vi "time_all_in_one.vi"(8 "Error In":errorcluster, 9 "Ship data?":bool, 10 "controls":T3={"window duration"=1.0, "width"=5, "crossing level"=0.0, "threshold"=0.25, "Sec"=1.0, "start time"=0.0} {"start time" format="%#_13g"; "Sec" format="%0.2f"; "threshold" format="%0.2f"; "crossing level" format="%#_13g"; "width" min=3; "window duration" format="%0.2f"}, 11 "waveform in":waveform(dbl)) -> (0 "Error out":errorcluster, 3 "time data cluster":T2)   [LabVIEW 2020]
uses:
  <vilib>/Waveform/WDTOps.llb/WDT Get Waveform Subset DBL.vi
  <vilib>/Analysis/1siggen.llb/Ramp Pattern by Delta.vi
  <vilib>/Analysis/NI_AALBase.lvlib
panel:
  out "XY Graph":T1(graph)
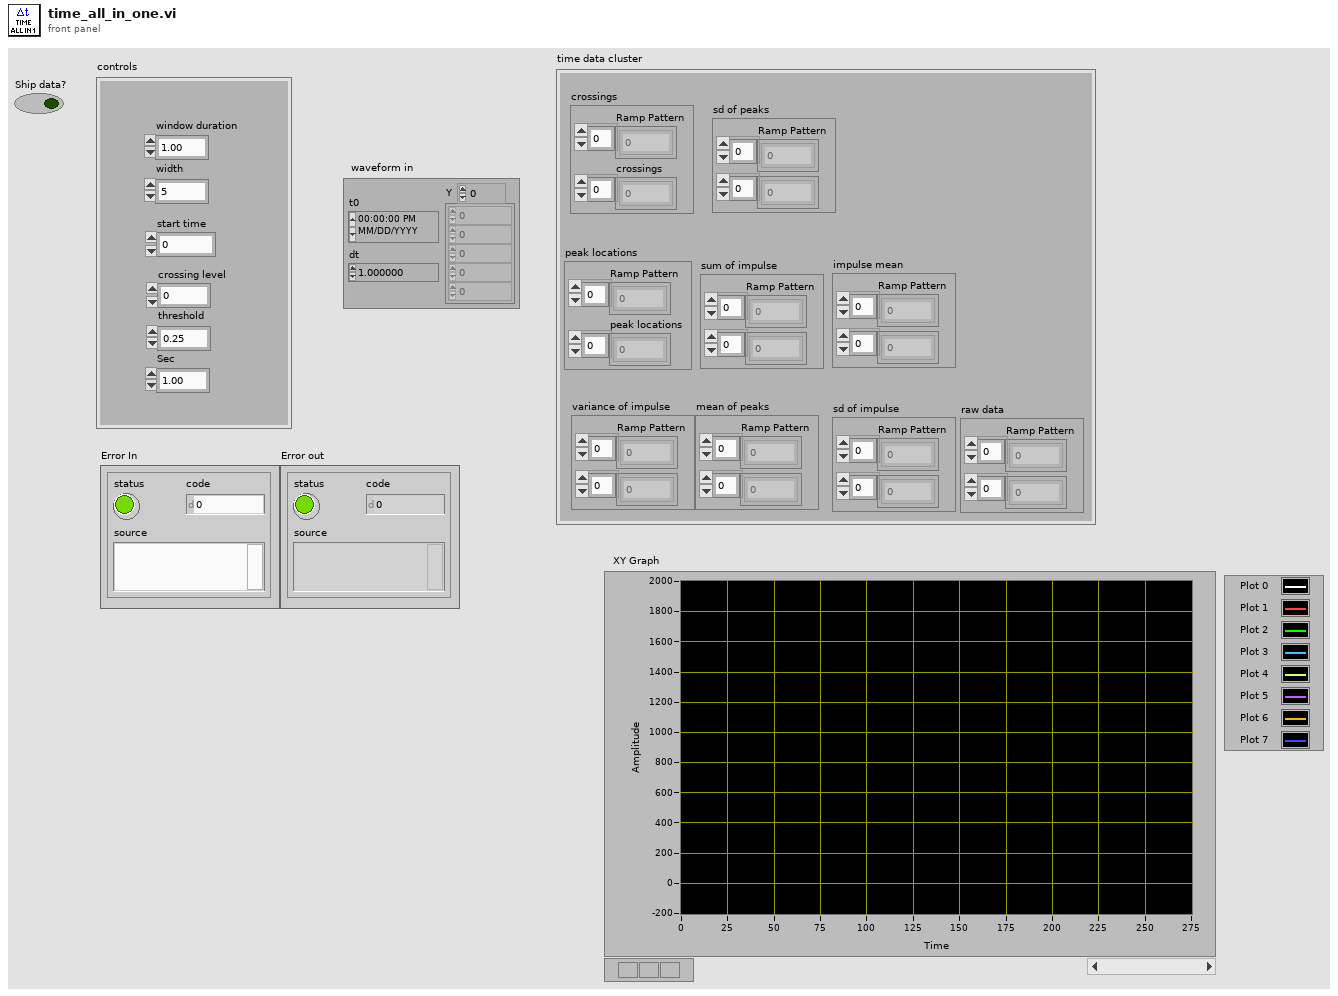
[diagram p1: front panel]
types:
  T1 = cluster{"Ramp Pattern":dbl[], "peak locations":dbl[]}[]
  T2 = cluster{"sd of peaks":cluster{"Ramp Pattern":dbl[], dbl[]}, "crossings":cluster{"Ramp Pattern":dbl[], "crossings":dbl[]}, "peak locations":cluster{"Ramp Pattern":dbl[], "peak locations":dbl[]}, "sum of impulse":cluster{"Ramp Pattern":dbl[], dbl[]}, "variance of impulse":cluster{"Ramp Pattern":dbl[], dbl[]}, "mean of peaks":cluster{"Ramp Pattern":dbl[], dbl[]}, "sd of impulse":cluster{"Ramp Pattern":dbl[], dbl[]}, "impulse mean":cluster{"Ramp Pattern":dbl[], dbl[]}, "raw data":cluster{"Ramp Pattern":dbl[], dbl[]}}
  T3 = cluster{"window duration":dbl, "width":i32, "crossing level":dbl, "threshold":dbl, "Sec":dbl, "start time":dbl}
  T4 = cluster{"Ramp Pattern":dbl[], "peak locations":dbl[]}
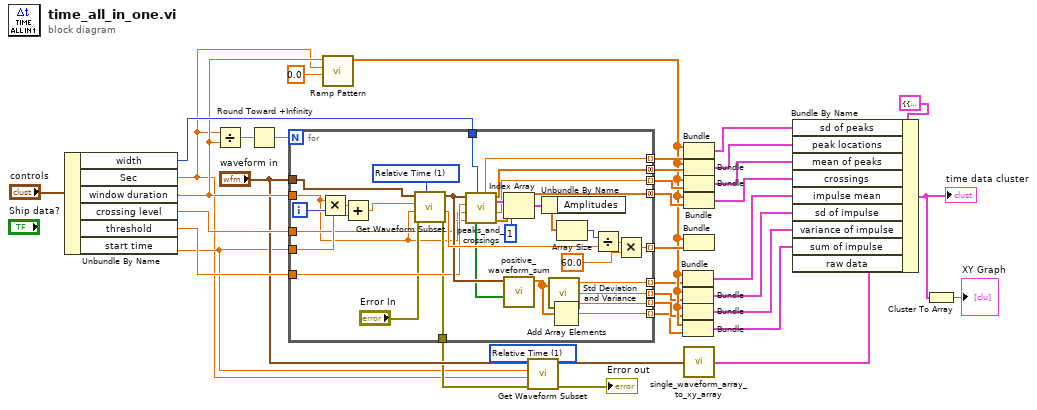
[diagram p0: block diagram]
diagram:
  w3 = u16 1 items=["Samples", "Relative Time"] ("start/duration format")
  n1 = Unbundle By Name("controls") -> ("width"=w34:i32, "Sec"=w1:dbl, "window duration"=w30:dbl, "crossing level"=w33:dbl, "threshold"=w32:dbl, "start time"=w2:dbl)
  n2 = Divide(x=w1, y=w30) -> (x/y=w37:dbl)
  n3 = Round Toward +Infinity(x=w37) -> (ceil(x): smallest int >= x=w36:dbl)
  n4 = for {
    N: w36 -> [_]
    tunnel: [w62] -> w25 mode=indexing
    tunnel: [w55] -> w22 mode=indexing
    tunnel: [w54] -> w20 mode=indexing
    tunnel: [w53] -> w23 mode=indexing
    tunnel: w30 -> [w38]
    tunnel: "waveform in" -> [w51]
    tunnel: w34 -> [w52]
    tunnel: w33 -> [w39]
    tunnel: w32 -> [w50]
    tunnel: [w49] -> w29 mode=indexing
    tunnel: [w48] -> w28 mode=concatenating
    tunnel: [w47] -> w27 mode=indexing
    tunnel: [w46] -> w26 mode=concatenating
    tunnel: [w45] -> w21 mode=indexing
    tunnel: w2 -> [w41]
    tunnel: [w43] -> w4
    i -> [w61]
    w59 = u16 1 items=["Samples", "Relative Time"] ("start/duration format")
    n5 = Multiply(x=w38, y=w61) -> (x*y=w42:dbl)
    n6 = Add(x=w42, y=w41) -> (x+y=w40:dbl)
    n7 = call-poly <vilib>:"Get Waveform Subset.vi"("start/duration format"=w59, "error in (no error)"="Error In", "duration"=w38, "start samples/time"=w40, "waveform in"=w51) -> ("error out"=w43:errorcluster, "actual duration"=w60:dbl, "waveform out"=w58:waveform(dbl))  [unwired: 1 in, 1 out]
    n8 = call "peaks_and_crossings.vi"("width"=w52, "crossing level"=w39, "end"=w38, "threshold"=w50, "waveform"=w58) -> ("crossings"=w46:dbl[], "mean of peaks"=w47:dbl, "all in array"=w69:cluster{dbl[], "Amplitudes":dbl[]}[], "peak locations"=w48:dbl[], "plus-minus crossing?"=w57:bool[], "standard deviation of peaks"=w49:dbl)  [unwired: 1 out]
    n9 = Index Array(array=w69, index=1) -> (element=w67:cluster{dbl[], "Amplitudes":dbl[]})
    n10 = call "positive_waveform_sum.vi"("plus-minus"=w57, "read in data"=w58) -> ("Integral X"=w56:dbl[])  [unwired: 8 in, 1 out]
    n11 = Unbundle By Name(w67) -> ("Amplitudes"=w66:dbl[])
    n12 = call <vilib>:"Std Deviation and Variance.vi"("X"=w56) -> ("mean"=w53:dbl, "standard deviation"=w55:dbl, "variance"=w45:dbl)  [unwired: 1 in]
    n13 = Add Array Elements(numeric array=w56) -> (sum=w54:dbl)
    n14 = Array Size(array=w66) -> (size(s)=w65:i32)
    n15 = Divide(x=w65, y=w60) -> (x/y=w64:dbl)
    n16 = Multiply(x=w64, y=60.0) -> (x*y=w62:dbl)
  }
  n17 = call-poly <vilib>:"Ramp Pattern.vi"("start"=0.0, "end"=w1, "delta"=w30) -> ("Ramp Pattern"=w24:dbl[])  [unwired: 6 in, 2 out]
  n18 = call-poly <vilib>:"Get Waveform Subset.vi"("start/duration format"=w3, "error in (no error)"=w4, "duration"=w1, "start samples/time"=w2, "waveform in"="waveform in") -> ("error out"=→"Error out":errorcluster, "waveform out"=w8:waveform(dbl))  [unwired: 1 in, 2 out]
  n19 = Bundle("Ramp Pattern"=w24, w23) -> (w15:cluster{"Ramp Pattern":dbl[], dbl[]})  [unwired: 1 in]
  n20 = Bundle("Ramp Pattern"=w24, w22) -> (w14:cluster{"Ramp Pattern":dbl[], dbl[]})  [unwired: 1 in]
  n21 = Bundle("Ramp Pattern"=w24, w21) -> (w13:cluster{"Ramp Pattern":dbl[], dbl[]})  [unwired: 1 in]
  n22 = Bundle("Ramp Pattern"=w24, w20) -> (w12:cluster{"Ramp Pattern":dbl[], dbl[]})  [unwired: 1 in]
  n23 = Bundle("Ramp Pattern"=w24, w29) -> (w19:cluster{"Ramp Pattern":dbl[], dbl[]})  [unwired: 1 in]
  n24 = Bundle("Ramp Pattern"=w24, "peak locations"=w28) -> (w18:T4)  [unwired: 1 in]
  n25 = Bundle("Ramp Pattern"=w24, w27) -> (w17:cluster{"Ramp Pattern":dbl[], dbl[]})  [unwired: 1 in]
  n26 = Bundle("Ramp Pattern"=w24, "crossings"=w26) -> (w16:cluster{"Ramp Pattern":dbl[], "crossings":dbl[]})  [unwired: 1 in]
  n27 = Bundle("Ramp Pattern"=w24, w25) -> ()  [unwired: 1 in, 1 out]
  n28 = call "single_waveform_array_to_xy_array.vi"("waveform in"=w8) -> ("XY out"=w6:cluster{dbl[], "Y":dbl[]})
  n29 = Bundle By Name(cluster=T2 {"sd of peaks"={"Ramp Pattern"=[0.0, 1.0], [0.11989676755880549]}, "crossings"={"Ramp Pattern"=[0.0, 1.0], "crossings"=[]}, "peak locations"={"Ramp Pattern"=[0.0, 1.0], "peak locations"=[0.03531286895522893, 0.09084899179766816, 0.1524822026967508, 0.22704874394974736, 0.3709465404161671, 0.5488212911270064]}, "sum of impulse"={"Ramp Pattern"=[0.0, 1.0], [0.0]}, "variance of impulse"={"Ramp Pattern"=[0.0, 1.0], [-0.0]}, "mean of peaks"={"Ramp Pattern"=[0.0, 1.0], [0.4789489584792137]}, "sd of impulse"={"Ramp Pattern"=[0.0, 1.0], [-0.0]}, "impulse mean"={"Ramp Pattern"=[0.0, 1.0], [nan]}, "raw data"={"Ramp Pattern"=[0.0, 1.0], [-0.0]}} ("time data cluster 2"), "sd of peaks"=w19, "peak locations"=w18, "mean of peaks"=w17, "crossings"=w16, "impulse mean"=w15, "sd of impulse"=w14, "variance of impulse"=w13, "sum of impulse"=w12, "raw data"=w6) -> (w10:T2)
  "time data cluster" <- w10
  n30 = Cluster To Array(cluster=w10) -> (array=→"XY Graph":T1)
